vi "Feedback.vi"(0 "time signal":waveform(dbl)) -> (1 "Result":dbl, 2 "x = y?":bool)   [LabVIEW 2013]
uses:
  <vilib>/measure/maspectr.llb/FFT Power Spectrum and PSD for 1 Chan.vi
  <vilib>/measure/NI_MAPro.lvlib
panel:
  out "df":dbl=2.2002200220022003 format="%#_6f"
  out "Amplitude (V)":dbl[](array[numeric])
  out "f0":dbl
  out "Waveform Graph":cluster{"f0":dbl, "df":dbl, "magnitude":dbl[]}(graph)
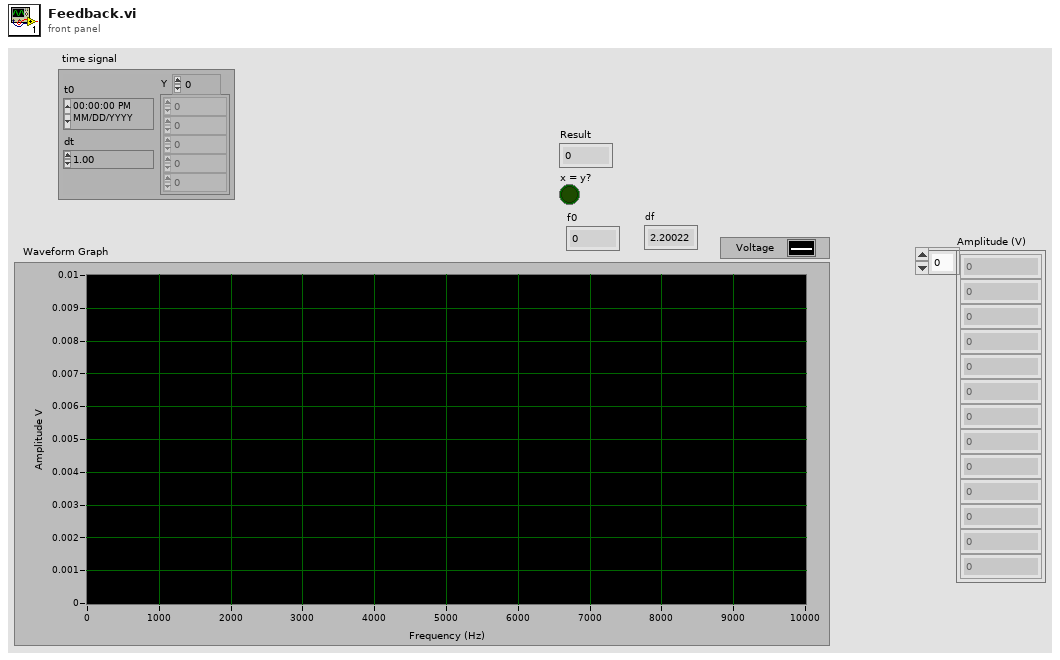
[diagram p1: front panel]
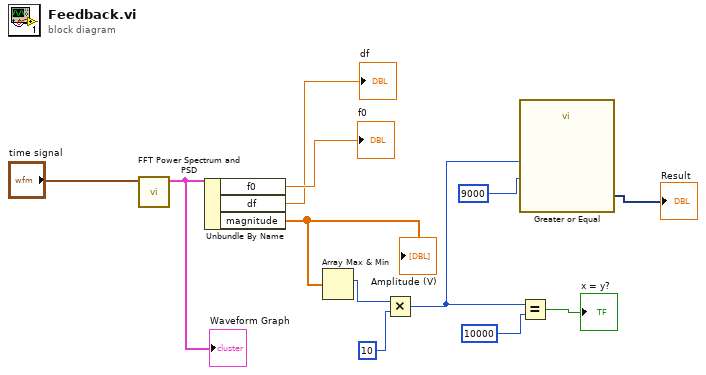
[diagram p0: block diagram]
diagram:
  n1 = call-poly <vilib>:"FFT Power Spectrum and PSD.vi"("time signal"="time signal") -> ("Power Spectrum / PSD"=w9:cluster{"f0":dbl, "df":dbl, "magnitude":dbl[]})  [unwired: 7 in, 3 out]
  "Waveform Graph" <- w9
  n2 = Unbundle By Name(w9) -> ("f0"=→"f0":dbl, "df"=→"df":dbl, "magnitude"=w10:dbl[])
  "Amplitude (V)" <- w10
  n3 = Array Max & Min(array=w10) -> (max index (indices)=w8:i32)  [unwired: 3 out]
  n4 = Multiply(x=w8, y=10) -> (x*y=w4:i32)
  n5 = call "Greater or Equal"("Constant Value to Compare Against"=9000, "Operand 1"=w4) -> ("Result"=→"Result":dynamicdata)  [unwired: 8 in, 1 out]
  n6 = Equal?(x=w4, y=10000) -> (x = y?=→"x = y?":bool)
